vi "Read XML_Parse BC Messages.vi"(8 "error in (no error)":errorcluster, 10 "channel in":T1, 11 ".NET Refnum in":refnum<k24>) -> (0 "error out":errorcluster, 2 "channel out":T1, 3 ".NET Refnum out":refnum<k24>)   [LabVIEW 2020, in "Ballard 1553 System Explorer.lvlib"]
uses:
  Ballard 1553 System Explorer.lvlib
  Ballard_Channel.ctl
  Ballard_BC.ctl
  Ballard_message.ctl
  Ballard_messageType.ctl
  Ballard_CWD1.ctl
  Ballard_CWD2.ctl
  Ballard_minorFrame.ctl
  Ballard_majorFrame.ctl
  Ballard_acyclicFrame.ctl
  Ballard_RT.ctl
  Ballard_RT subAddress.ctl
  Ballard_RT direction.ctl
  Ballard_RT rtMode.ctl
  Ballard_RT modeCode.ctl
  C:/Users/Administrator/Desktop/GIT/Ballard-MIL-STD-1553-Custom-Device/Source/System Explorer/SubVIs/Parse XML Ballard/Ballard_BTI_XML_MIL_STD_1553_Deserializer.dll
  Ballard_BTI_XML_MIL_STD_1553_Deserializer.dll
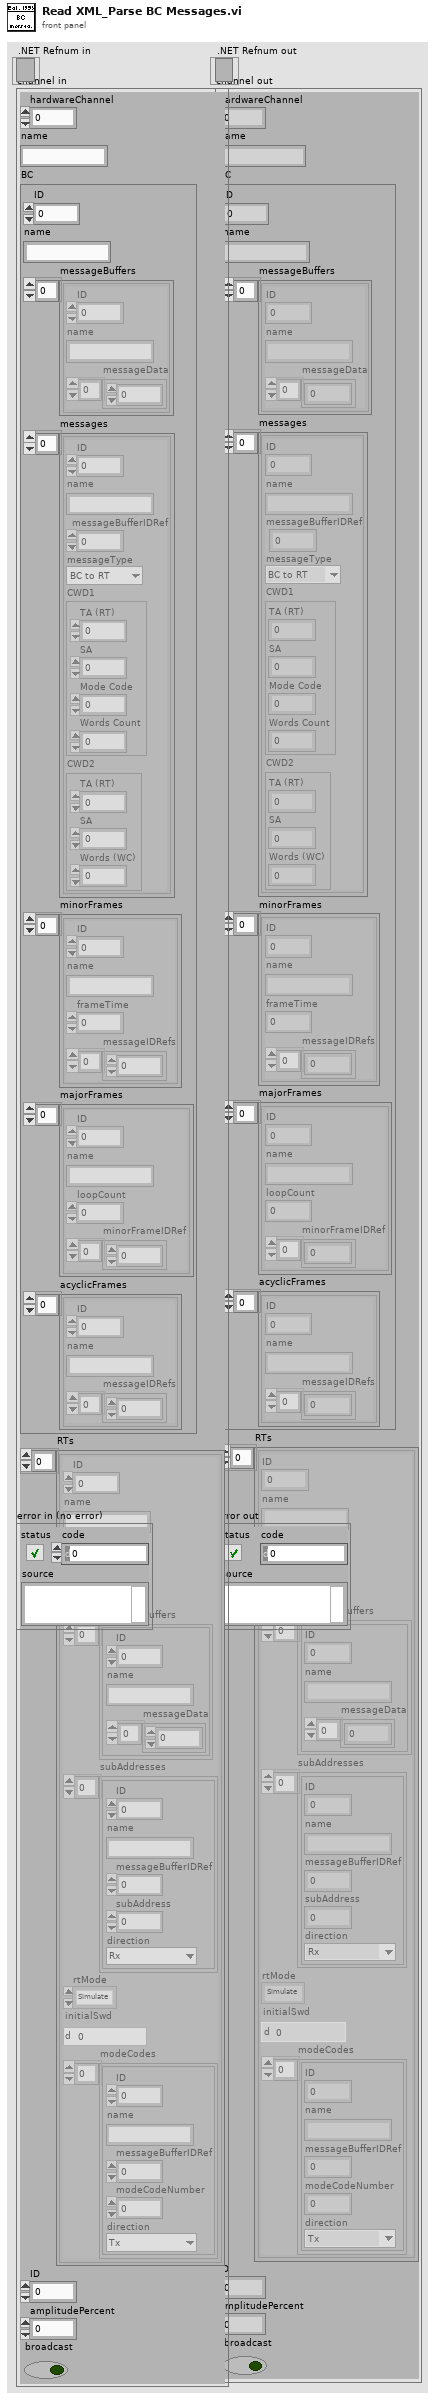
[diagram p1: front panel]
types:
  T1 = typedef "Ballard 1553 System Explorer.lvlib/Ballard_Channel.ctl" = cluster{"hardwareChannel":i32, "name":string, "BC":T2, "RTs":T10[], "ID":i32, "amplitudePercent":dbl, "broadcast":bool}
  T2 = typedef "Ballard 1553 System Explorer.lvlib/Ballard_BC.ctl" = cluster{"ID":i32, "name":string, "messageBuffers":cluster{"ID":i32, "name":string, "messageData":u16[]}[], "messages":T3[], "minorFrames":T7[], "majorFrames":T8[], "acyclicFrames":T9[]}
  T3 = typedef "Ballard 1553 System Explorer.lvlib/Ballard_message.ctl" = cluster{"ID":i32, "name":string, "messageBufferIDRef":i32, "messageType":T4, "CWD1":T5, "CWD2":T6}
  T4 = typedef "Ballard 1553 System Explorer.lvlib/Ballard_messageType.ctl" = enum16{"BC to RT", "RT to BC", "RT to RT", "MC (Rx)", "MC (Tx)"}
  T5 = typedef "Ballard 1553 System Explorer.lvlib/Ballard_CWD1.ctl" = cluster{"TA (RT)":i8, "SA":i8, "Mode Code":i8, "Words Count":i8}
  T6 = typedef "Ballard 1553 System Explorer.lvlib/Ballard_CWD2.ctl" = cluster{"TA (RT)":i8, "SA":i8, "Words (WC)":i8}
  T7 = typedef "Ballard 1553 System Explorer.lvlib/Ballard_minorFrame.ctl" = cluster{"ID":i32, "name":string, "frameTime":i32, "messageIDRefs":i32[]}
  T8 = typedef "Ballard 1553 System Explorer.lvlib/Ballard_majorFrame.ctl" = cluster{"ID":i32, "name":string, "loopCount":i32, "minorFrameIDRef":i32[]}
  T9 = typedef "Ballard 1553 System Explorer.lvlib/Ballard_acyclicFrame.ctl" = cluster{"ID":i32, "name":string, "messageIDRefs":i32[]}
  T10 = typedef "Ballard 1553 System Explorer.lvlib/Ballard_RT.ctl" = cluster{"ID":i32, "name":string, "rtAddress":i8, "responseTime":i32, "messageBuffers":cluster{"ID":i32, "name":string, "messageData":u16[]}[], "subAddresses":T11[], "rtMode":T13, "initialSwd":u16, "modeCodes":T14[]}
  T11 = typedef "Ballard 1553 System Explorer.lvlib/Ballard_RT subAddress.ctl" = cluster{"ID":i32, "name":string, "messageBufferIDRef":i32, "subAddress":i8, "direction":T12}
  T12 = typedef "Ballard 1553 System Explorer.lvlib/Ballard_RT direction.ctl" = enum16{"Tx", "Rx"}
  T13 = typedef "Ballard 1553 System Explorer.lvlib/Ballard_RT rtMode.ctl" = enum16{"Simulate", "Monitor", "Disable"}
  T14 = typedef "Ballard 1553 System Explorer.lvlib/Ballard_RT modeCode.ctl" = cluster{"ID":i32, "name":string, "messageBufferIDRef":i32, "modeCodeNumber":i8, "direction":T12}
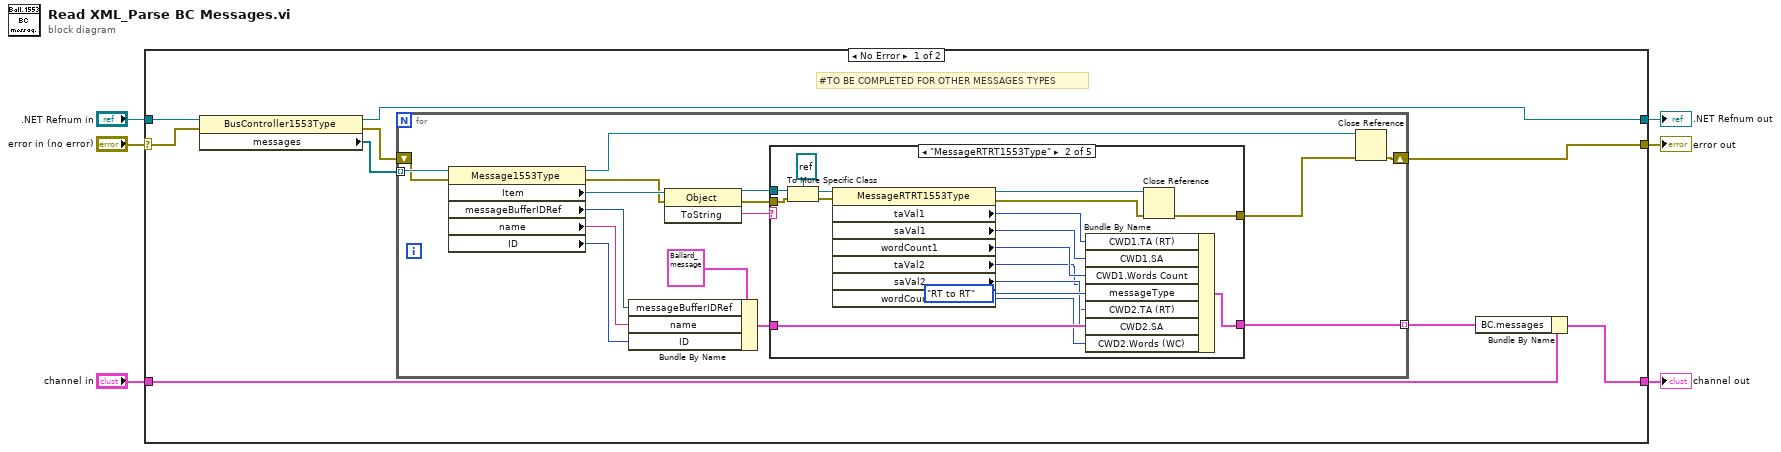
[diagram p0: block diagram]
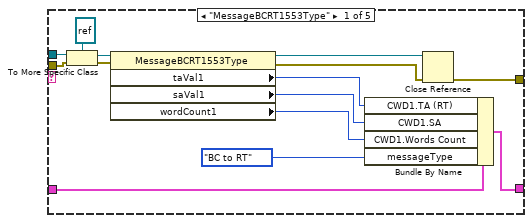
[diagram p2: hidden frame]
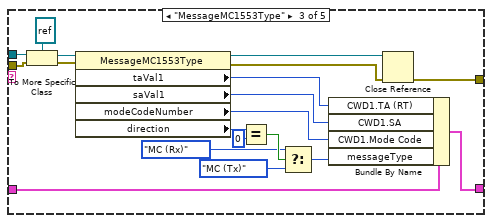
[diagram p3: hidden frame]
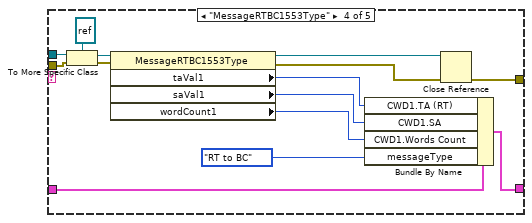
[diagram p4: hidden frame]
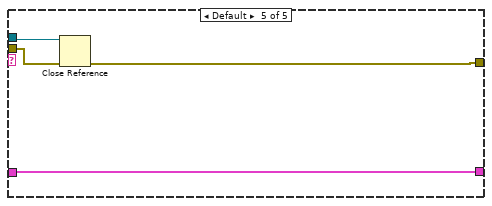
[diagram p5: hidden frame]
diagram:
  n1 = case shown="No Error" "error in (no error)" {
    selector: "error in (no error)" -> [w7 w101]
    tunnel: [w15 w100] -> w6
    tunnel: [w14 w102] -> w5
    tunnel: [w13 w101] -> w4
    tunnel: "channel in" -> [w10 w100]
    tunnel: ".NET Refnum in" -> [w8 w102]
    frame No Error {
      # "#TO BE COMPLETED FOR OTHER MESSAGES TYPES"
      n2 = property class="BusController1553Type"(reference=w8, error in=w7) -> (reference out=w14:refnum<k24>, error out=w11:errorcluster, "messages"=w9:refnum<k24>[])
      n3 = for {
        tunnel: w9 -> [w31] mode=indexing
        shift-right: [w28] -> w13
        shift-left: w11 -> [w30]
        tunnel: [w17] -> w12 mode=indexing
        n4 = property class="Message1553Type"(reference=w31, error in=w30) -> (reference out=w29:refnum<k24>, error out=w22:errorcluster, "Item"=w26:refnum<k24>, "messageBufferIDRef"=w23:i32, "name"=w24:string, "ID"=w27:i32)
        n5 = Bundle By Name(cluster=T3 {"ID"=0, "name"="", "messageBufferIDRef"=0, "messageType"=enum."BC to RT", "CWD1"={"TA (RT)"=0, "SA"=0, "Mode Code"=0, "Words Count"=0}, "CWD2"={"TA (RT)"=0, "SA"=0, "Words (WC)"=0}} ("message"), "messageBufferIDRef"=w23, "name"=w24, "ID"=w27) -> (w18:T3)
        n6 = invoke class="Object" method="ToString"(reference=w26, error in=w22) -> (reference out=w21:refnum<k24>, error out=w20:errorcluster, "ToString"=w19:string)  [unwired: 1 in]
        n7 = case shown="\"MessageRTRT1553Type\"" w19 {
          tunnel: w21 -> [w44 w61 w80 w94 w99]
          tunnel: w20 -> [w43 w60 w79 w93 w98]
          tunnel: w18 -> [w40 w57 w76 w90 w96]
          tunnel: [w35 w52 w73 w85 w96] -> w17
          tunnel: [w32 w49 w70 w82 w97] -> w16
          frame "MessageBCRT1553Type" {
            n8 = To More Specific Class(target class=refnum<k24> refnum, reference=w44, error in=w43) -> (specific class reference=w41:refnum<k24>, error out=w42:errorcluster)
            n9 = property class="MessageBCRT1553Type"(reference=w41, error in=w42) -> (reference out=w33:refnum<k24>, error out=w34:errorcluster, "taVal1"=w38:i8, "saVal1"=w37:i8, "wordCount1"=w36:i8)
            n10 = Bundle By Name(cluster=w40, "CWD1.TA (RT)"=w38, "CWD1.SA"=w37, "CWD1.Words Count"=w36, "messageType"=Ballard_messageType."BC to RT") -> (w35:T3)
            n11 = Close Reference(reference=w33, error in (no error)=w34) -> (error out=w32:errorcluster)
          }
          frame "MessageRTRT1553Type" {
            n12 = To More Specific Class(target class=refnum<k24> refnum, reference=w61, error in=w60) -> (specific class reference=w58:refnum<k24>, error out=w59:errorcluster)
            n13 = property class="MessageRTRT1553Type"(reference=w58, error in=w59) -> (reference out=w50:refnum<k24>, error out=w51:errorcluster, "taVal1"=w55:i8, "saVal1"=w54:i8, "wordCount1"=w53:i8, "taVal2"=w46:i8, "saVal2"=w47:i8, "wordCount2"=w48:i8)
            n14 = Bundle By Name(cluster=w57, "CWD1.TA (RT)"=w55, "CWD1.SA"=w54, "CWD1.Words Count"=w53, "messageType"=Ballard_messageType."RT to RT", "CWD2.TA (RT)"=w46, "CWD2.SA"=w47, "CWD2.Words (WC)"=w48) -> (w52:T3)
            n15 = Close Reference(reference=w50, error in (no error)=w51) -> (error out=w49:errorcluster)
          }
          frame "MessageMC1553Type" {
            n16 = To More Specific Class(target class=refnum<k24> refnum, reference=w80, error in=w79) -> (specific class reference=w77:refnum<k24>, error out=w78:errorcluster)
            n17 = property class="MessageMC1553Type"(reference=w77, error in=w78) -> (reference out=w71:refnum<k24>, error out=w72:errorcluster, "taVal1"=w75:i8, "saVal1"=w74:i8, "modeCodeNumber"=w69:i8, "direction"=w67:i32)
            n18 = Equal?(x=w67, y=0) -> (x = y?=w68:bool)
            n19 = Select(t=Ballard_messageType."MC (Rx)" ("messageType"), s=w68, f=Ballard_messageType."MC (Tx)") -> (s? t:f=w63:T4)
            n20 = Bundle By Name(cluster=w76, "CWD1.TA (RT)"=w75, "CWD1.SA"=w74, "CWD1.Mode Code"=w69, "messageType"=w63) -> (w73:T3)
            n21 = Close Reference(reference=w71, error in (no error)=w72) -> (error out=w70:errorcluster)
          }
          frame "MessageRTBC1553Type" {
            n22 = To More Specific Class(target class=refnum<k24> refnum, reference=w94, error in=w93) -> (specific class reference=w91:refnum<k24>, error out=w92:errorcluster)
            n23 = property class="MessageRTBC1553Type"(reference=w91, error in=w92) -> (reference out=w83:refnum<k24>, error out=w84:errorcluster, "taVal1"=w88:i8, "saVal1"=w87:i8, "wordCount1"=w86:i8)
            n24 = Bundle By Name(cluster=w90, "CWD1.TA (RT)"=w88, "CWD1.SA"=w87, "CWD1.Words Count"=w86, "messageType"=Ballard_messageType."RT to BC") -> (w85:T3)
            n25 = Close Reference(reference=w83, error in (no error)=w84) -> (error out=w82:errorcluster)
          }
          frame Default {
            n26 = Close Reference(reference=w99, error in (no error)=w98) -> (error out=w97:errorcluster)
          }
        }
        n27 = Close Reference(reference=w29, error in (no error)=w16) -> (error out=w28:errorcluster)
      }
      n28 = Bundle By Name(cluster=w10, "BC.messages"=w12) -> (w15:T1)
    }
    frame Error {
    }
  }
  "channel out" <- w6
  ".NET Refnum out" <- w5
  "error out" <- w4
